vi "poly_linspace_CSG.vi"(6 "inclusive? (T)":bool=TRUE, 7 "mode (cartesian)":T1(ring), 8 "xN":csg, 9 "N":i32, 10 "x0":csg) -> (1 "linspace out":csg[](array[numeric]))   [LabVIEW 2015]
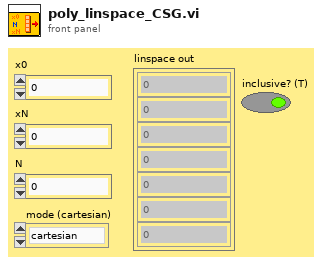
[diagram p1: front panel]
types:
  T1 = enum16{"cartesian", "angular (+)", "angular (-)"}
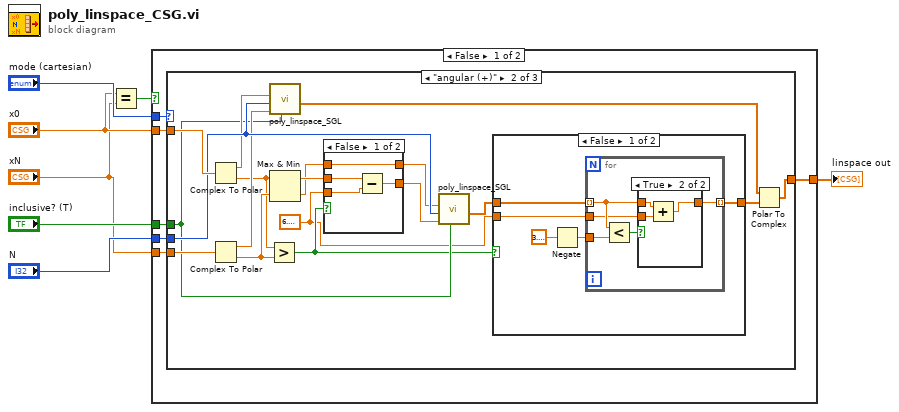
[diagram p0: block diagram]
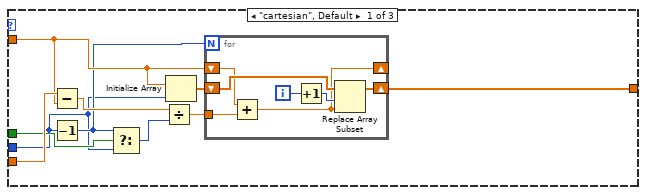
[diagram p2: hidden frame]
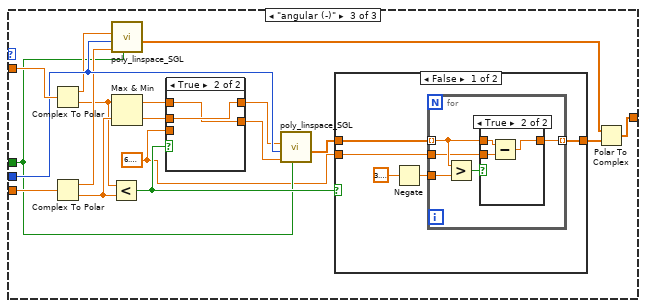
[diagram p6: hidden frame]
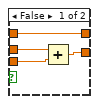
[diagram p9: hidden frame]
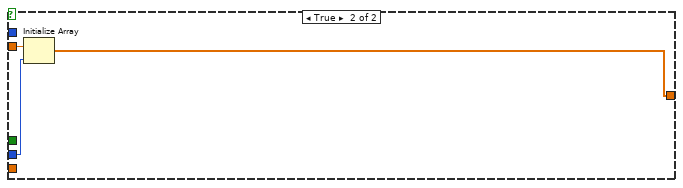
[diagram p10: hidden frame]
diagram:
  n1 = Equal?(x="x0", y="xN") -> (x = y?=w1:bool)
  n2 = case shown="False" w1 {
    tunnel: "xN" -> [w13 _]
    tunnel: "x0" -> [w12 w111]
    tunnel: "inclusive? (T)" -> [w11 _]
    tunnel: "N" -> [w10 w110]
    tunnel: [w9 w109] -> w5
    tunnel: "mode (cartesian)" -> [w8 _]
    frame False {
      n3 = case shown="\"angular (+)\"" w8 {
        tunnel: [w22 w44 w83] -> w9
        tunnel: w13 -> [w21 w47 w86]
        tunnel: w12 -> [w20 w48 w87]
        tunnel: w11 -> [w18 w38 w71]
        tunnel: w10 -> [w14 w46 w85]
        frame "cartesian", Default {
          n4 = Subtract(x=w21, y=w20) -> (x-y=w16:csg)
          n5 = Decrement(x=w14) -> (x-1=w15:i32)
          n6 = Select(t=w15, s=w18, f=w14) -> (s? t:f=w17:i32)
          n7 = Divide(x=w16, y=w17) -> (x/y=w19:csg)
          n8 = Initialize Array(w20, w14) -> (w23:csg[])
          n9 = for {
            N: w15 -> [_]
            shift-right: [w27] -> w22
            shift-left: w23 -> [w30]
            shift-right: [w24] -> _
            shift-left: w20 -> [w29]
            tunnel: w19 -> [w28]
            i -> [w26]
            n10 = Add(x=w29, y=w28) -> (x+y=w24:csg)
            n11 = Increment(x=w26) -> (x+1=w25:i32)
            n12 = Replace Array Subset(array=w30, new element=w24, index=w25) -> (w27:csg[])
          }
        }
        frame "angular (+)" {
          w31 = sgl 6.2831855
          n13 = Complex To Polar(r * e^(i*theta)=w48) -> (r=w43:sgl, theta=w39:sgl)
          n14 = Complex To Polar(r * e^(i*theta)=w47) -> (r=w42:sgl, theta=w40:sgl)
          n15 = Greater?(x=w39, y=w40) -> (0:w32:bool)
          n16 = call "poly_linspace_SGL.vi"("inclusive? (T)"=w38, "xN"=w42, "N"=w46, "x0"=w43) -> ("linspace out"=w45:sgl[])  [unwired: 7 in]
          n17 = Max & Min(x=w39, y=w40) -> (max(x,y)=w37:sgl, min(x,y)=w34:sgl)
          n18 = case shown="False" w32 {
            tunnel: w37 -> [w66 w69]
            tunnel: [w67 w69] -> w36
            tunnel: [w65 w68] -> w35
            tunnel: w34 -> [w67 w68]
            tunnel: w31 -> [w64 _]
            frame False {
              n19 = Subtract(x=w66, y=w64) -> (x-y=w65:sgl)
            }
            frame True {
            }
          }
          n20 = call "poly_linspace_SGL.vi"("inclusive? (T)"=w38, "xN"=w35, "N"=w46, "x0"=w36) -> ("linspace out"=w33:sgl[])  [unwired: 7 in]
          n21 = case shown="False" w32 {
            tunnel: [w52 w63] -> w41
            tunnel: w33 -> [w53 w63]
            tunnel: w31 -> [w51 _]
            frame False {
              n22 = Negate(x=sgl 3.1415927) -> (-x=w49:sgl)
              n23 = for {
                tunnel: w53 -> [w56] mode=indexing
                tunnel: [w57] -> w52 mode=indexing
                tunnel: w51 -> [w55]
                tunnel: w49 -> [w54]
                n24 = Less?(x=w56, y=w54) -> (x < y?=w58:bool)
                n25 = case shown="True" w58 {
                  tunnel: [w59 w60] -> w57
                  tunnel: w56 -> [w59 w62]
                  tunnel: w55 -> [_ w61]
                  frame False {
                  }
                  frame True {
                    n26 = Add(x=w62, y=w61) -> (x+y=w60:sgl)
                  }
                }
              }
            }
            frame True {
            }
          }
          n27 = Polar To Complex(1:w41, 2:w45) -> (0:w44:csg[])
        }
        frame "angular (-)" {
          w70 = sgl 6.2831855
          n28 = Complex To Polar(r * e^(i*theta)=w87) -> (r=w82:sgl, theta=w78:sgl)
          n29 = Complex To Polar(r * e^(i*theta)=w86) -> (r=w81:sgl, theta=w79:sgl)
          n30 = Less?(x=w78, y=w79) -> (x < y?=w72:bool)
          n31 = call "poly_linspace_SGL.vi"("inclusive? (T)"=w71, "xN"=w81, "N"=w85, "x0"=w82) -> ("linspace out"=w84:sgl[])  [unwired: 7 in]
          n32 = Max & Min(x=w78, y=w79) -> (max(x,y)=w77:sgl, min(x,y)=w74:sgl)
          n33 = case shown="True" w72 {
            tunnel: w77 -> [w104 w107]
            tunnel: [w104 w108] -> w76
            tunnel: [w106 w107] -> w75
            tunnel: w74 -> [w103 w108]
            tunnel: w70 -> [w105 _]
            frame False {
              n34 = Add(x=w103, y=w105) -> (x+y=w106:sgl)
            }
            frame True {
            }
          }
          n35 = call "poly_linspace_SGL.vi"("inclusive? (T)"=w71, "xN"=w75, "N"=w85, "x0"=w76) -> ("linspace out"=w73:sgl[])  [unwired: 7 in]
          n36 = case shown="False" w72 {
            tunnel: [w91 w102] -> w80
            tunnel: w73 -> [w92 w102]
            tunnel: w70 -> [w90 _]
            frame False {
              n37 = Negate(x=sgl 3.1415927) -> (-x=w88:sgl)
              n38 = for {
                tunnel: w92 -> [w95] mode=indexing
                tunnel: [w96] -> w91 mode=indexing
                tunnel: w90 -> [w94]
                tunnel: w88 -> [w93]
                n39 = Greater?(x=w95, y=w93) -> (0:w97:bool)
                n40 = case shown="True" w97 {
                  tunnel: [w98 w99] -> w96
                  tunnel: w95 -> [w98 w101]
                  tunnel: w94 -> [_ w100]
                  frame False {
                  }
                  frame True {
                    n41 = Subtract(x=w101, y=w100) -> (x-y=w99:sgl)
                  }
                }
              }
            }
            frame True {
            }
          }
          n42 = Polar To Complex(1:w80, 2:w84) -> (0:w83:csg[])
        }
      }
    }
    frame True {
      n43 = Initialize Array(w111, w110) -> (w109:csg[])
    }
  }
  "linspace out" <- w5
